vi "Reload Previous Command.vi"(6 "Front (T) Back (F)":bool, 8 "error in (no error)":errorcluster, 10 "index":i32, 11 "Command Handler in":refnum<class "Command Handler.lvclass">) -> (0 "error out":errorcluster, 3 "Command Handler out":refnum<class "Command Handler.lvclass">)   [LabVIEW 2017, in "Command Handler.lvlib" / "Command Handler.lvclass"]
uses:
  Command Handler.lvclass
  Command Handler.lvclass/Command Handler.ctl
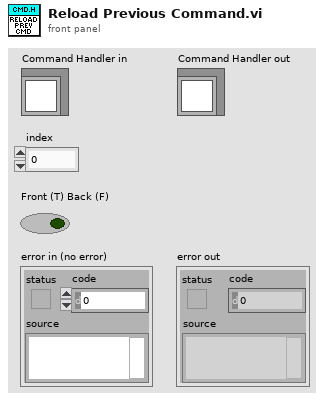
[diagram p1: front panel]
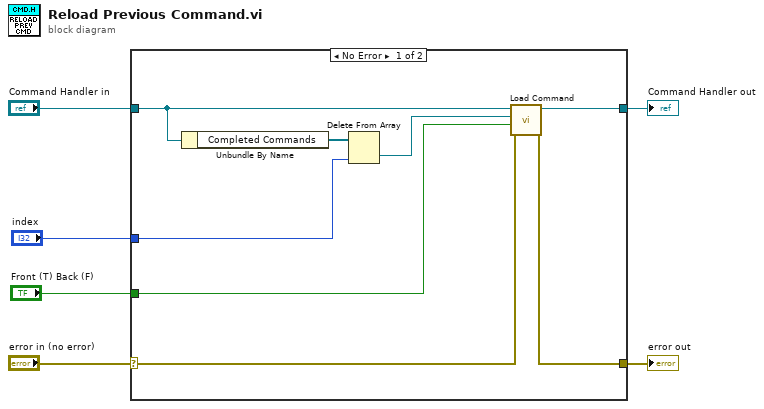
[diagram p0: block diagram]
diagram:
  n1 = case shown="No Error" "error in (no error)" {
    selector: "error in (no error)" -> [w10 w16]
    tunnel: [w9 w16] -> w5
    tunnel: [w11 w15] -> w3
    tunnel: "Command Handler in" -> [w12 w15]
    tunnel: "index" -> [w13 _]
    tunnel: "Front (T) Back (F)" -> [w7 _]
    frame No Error {
      n2 = Unbundle By Name(w12) -> ("Completed Commands"=w14:refnum<class "Command.lvclass">[])
      n3 = Delete From Array(array=w14, index=w13) -> (deleted portion=w8:refnum<class "Command.lvclass">)  [unwired: 1 in, 1 out]
      n4 = call-dynamic "Load Command.vi"("error in (no error)"=w10, "Front (T) Back (F)"=w7, "Command In"=w8, "Command Handler in"=w12) -> ("error out"=w9:errorcluster, "Command Handler out"=w11:refnum<class "Command Handler.lvclass">)  [unwired: 6 in]
    }
    frame Error {
    }
  }
  "error out" <- w5
  "Command Handler out" <- w3
